vi "Write Config file.vi"(8 "error in (no error)":errorcluster, 10 "Config file":path, 11 "Lamp Container in":refnum<class "Lamp Container.lvclass">) -> (0 "error out":errorcluster, 3 "Lamp Container out":refnum<class "Lamp Container.lvclass">)   [LabVIEW 2016, in "Lamp Container.lvclass"]
uses:
  Lamp Container.lvclass
  Lamp Container.lvclass/Lamp Container.ctl
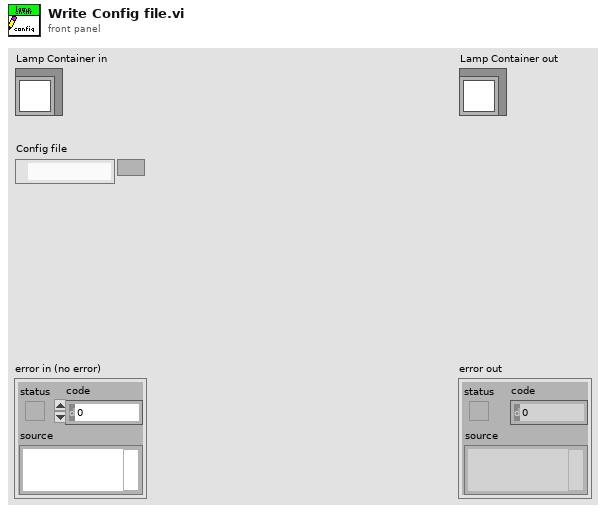
[diagram p1: front panel]
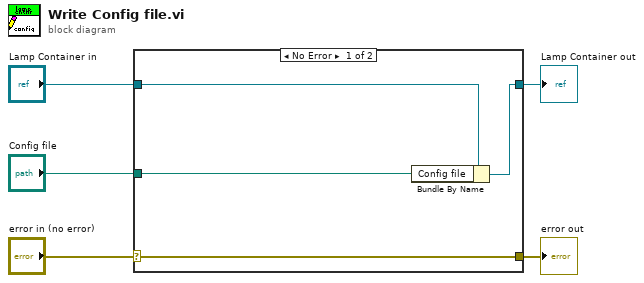
[diagram p0: block diagram]
diagram:
  n1 = case shown="No Error" "error in (no error)" {
    selector: "error in (no error)" -> [w9 w10]
    tunnel: [w9 w10] -> w4
    tunnel: [w7 w11] -> w2
    tunnel: "Lamp Container in" -> [w8 w11]
    tunnel: "Config file" -> [w6 _]
    frame No Error {
      n2 = Bundle By Name(cluster=w8, "Config file"=w6) -> (w7:refnum<class "Lamp Container.lvclass">)
    }
    frame Error {
    }
  }
  "error out" <- w4
  "Lamp Container out" <- w2
